vi "Decimate.vi"(1 "i":i32, 2 "n":i32, 3 "Input Array":u32[](array[numeric])) -> (0 "Decimated Array":u32[](array[numeric]))   [LabVIEW 2014]
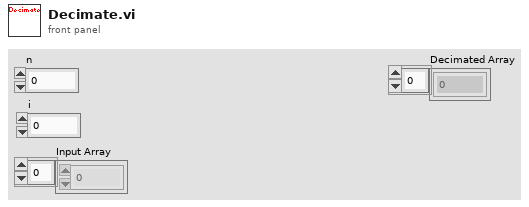
[diagram p1: front panel]
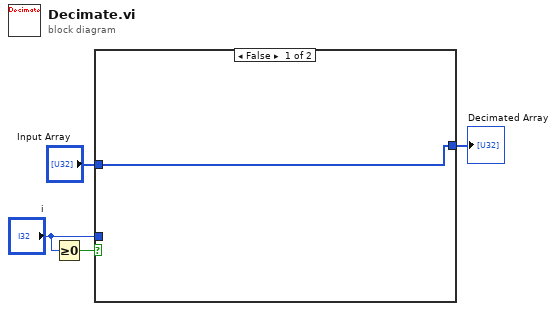
[diagram p0: block diagram]
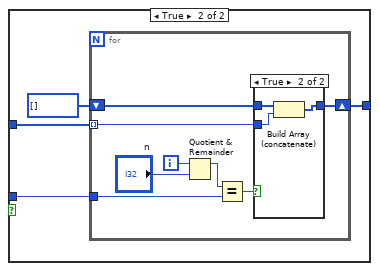
[diagram p2: hidden frame]
diagram:
  n1 = Greater Or Equal To 0?(x="i") -> (x >= 0?=w1:bool)
  n2 = case shown="False" w1 {
    tunnel: [w5 w8] -> w4
    tunnel: "Input Array" -> [w5 w7]
    tunnel: "i" -> [_ w6]
    frame False {
    }
    frame True {
      n3 = for {
        shift-right: [w14] -> w8
        shift-left: u32[] [] -> [w15]
        tunnel: w7 -> [w11] mode=indexing
        tunnel: w6 -> [w10]
        i -> [w13]
        n4 = Quotient & Remainder(x=w13, y="n") -> (x-y*floor(x/y)=w17:i32)  [unwired: 1 out]
        n5 = Equal?(x=w17, y=w10) -> (x = y?=w16:bool)
        n6 = case shown="True" w16 {
          tunnel: [w18 w21] -> w14
          tunnel: w15 -> [w18 w20]
          tunnel: w11 -> [_ w19]
          frame False {
          }
          frame True {
            n7 = Build Array (concatenate)(w20, w19) -> (w21:u32[])
          }
        }
      }
    }
  }
  "Decimated Array" <- w4
